vi "First Existing Folder in Path.vi"(11 "Stripped Path In":path) -> (3 "Stripped Path Out":path)   [LabVIEW 2017, in "CSM File Logger.lvlib"]
uses:
  CSM File Logger.lvlib
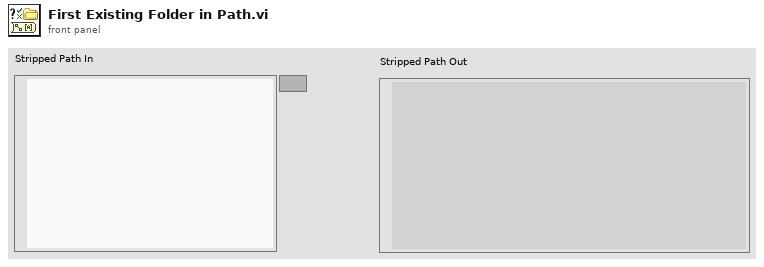
[diagram p1: front panel]
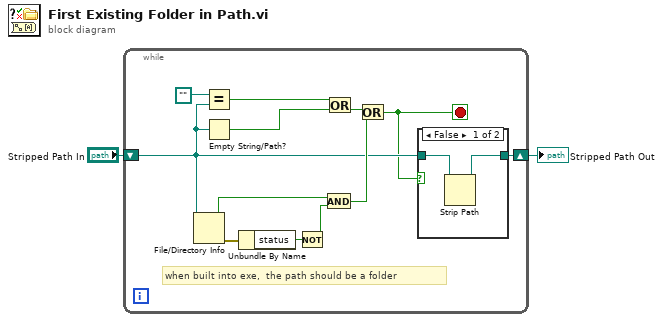
[diagram p0: block diagram]
diagram:
  n1 = while {
    shift-right: [w4] -> w2
    shift-left: "Stripped Path In" -> [w5]
    stop <- w3 stop-if-true
    # "when built into exe,  the path should be a folder"
    n2 = File/Directory Info(path=w5) -> (directory=w10:bool, error out=w6:errorcluster)  [unwired: 1 in, 5 out]
    n3 = Equal?(x=path "", y=w5) -> (x = y?=w12:bool)
    n4 = Empty String/Path?(string/path=w5) -> (empty?=w14:bool)
    n5 = Unbundle By Name(w6) -> ("status"=w7:bool)
    n6 = Not(x=w7) -> (.not. x?=w9:bool)
    n7 = And(x=w10, y=w9) -> (x .and. y?=w8:bool)
    n8 = Or(x=w12, y=w14) -> (x .or. y?=w13:bool)
    n9 = Or(x=w13, y=w8) -> (x .or. y?=w3:bool)
    n10 = case shown="False" w3 {
      tunnel: w5 -> [w16 w17]
      tunnel: [w15 w17] -> w4
      frame False {
        n11 = Strip Path(path=w16) -> (stripped path=w15:path)  [unwired: 1 out]
      }
      frame True {
      }
    }
  }
  "Stripped Path Out" <- w2
